vi "Write Sim Speed.vi"(8 "error in (no error)":errorcluster, 10 "Sim Speed":refnum<data-value>, 11 "Pump.Simulated in":refnum<class "Pump.Simulated.lvclass">) -> (0 "error out":errorcluster, 3 "Pump.Simulated out":refnum<class "Pump.Simulated.lvclass">)   [LabVIEW 2014, in "Pump.Simulated.lvclass"]
uses:
  Pump.Simulated.lvclass
  Pump.Simulated.lvclass/Pump.Simulated.ctl
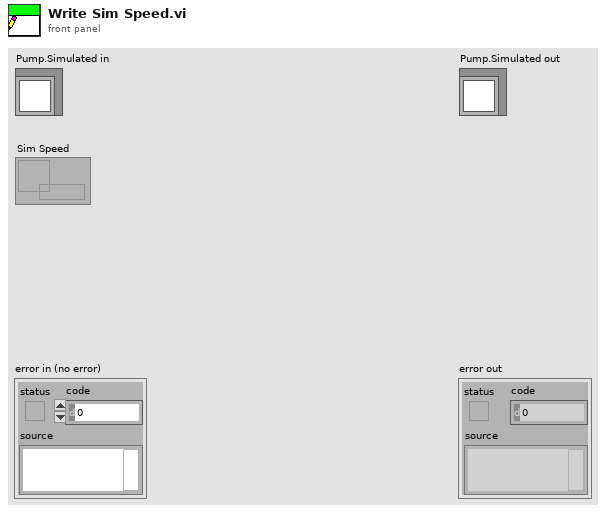
[diagram p1: front panel]
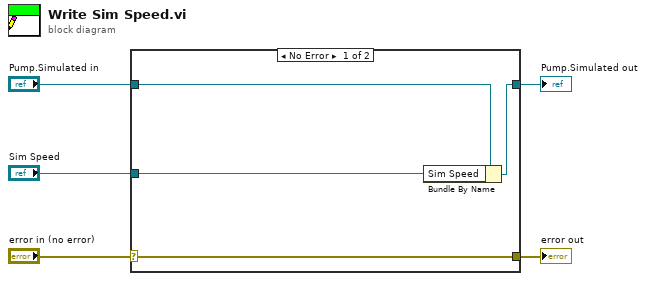
[diagram p0: block diagram]
diagram:
  n1 = case shown="No Error" "error in (no error)" {
    selector: "error in (no error)" -> [w9 w10]
    tunnel: [w9 w10] -> w4
    tunnel: [w7 w11] -> w2
    tunnel: "Pump.Simulated in" -> [w8 w11]
    tunnel: "Sim Speed" -> [w6 _]
    frame No Error {
      n2 = Bundle By Name(cluster=w8, "Sim Speed"=w6) -> (w7:refnum<class "Pump.Simulated.lvclass">)
    }
    frame Error {
    }
  }
  "error out" <- w4
  "Pump.Simulated out" <- w2
